vi "ABB change password.vi"() -> ()   [LabVIEW 2017]
uses:
  ABB global.vi
panel:
  out "Message":string
  in  "OK":bool
  in  "Cancel":bool
  in  "Confirm":string
  in  "New Password":string
  # "CHANGE PASSWORD"
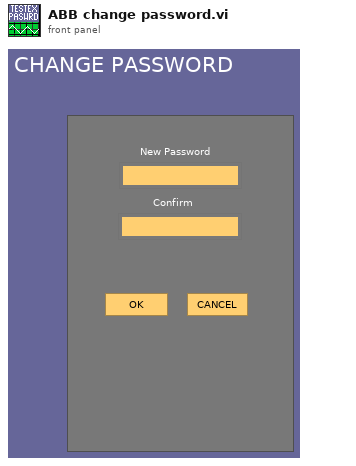
[diagram p1: front panel]
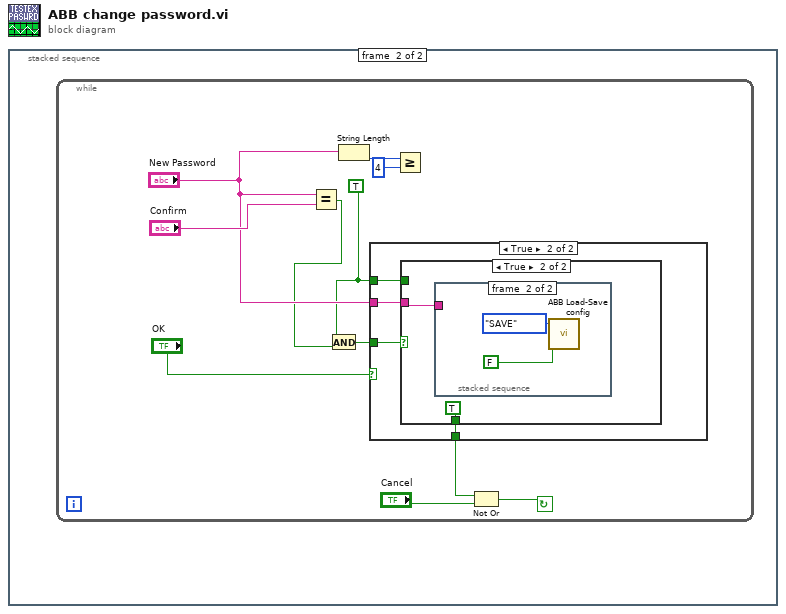
[diagram p0: block diagram]
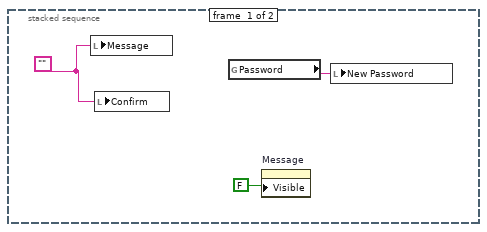
[diagram p2: hidden frame]
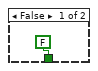
[diagram p3: hidden frame]
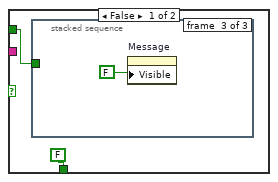
[diagram p4: hidden frame]
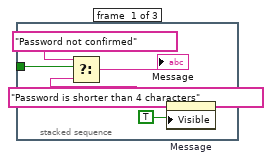
[diagram p5: hidden frame]
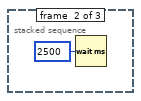
[diagram p6: hidden frame]
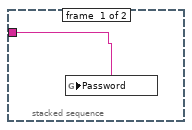
[diagram p7: hidden frame]
diagram:
  n1 = stacked-sequence {
    frame #0 {
      w2 = ""
      n2 = local write "Message"(w2) -> ()
      n3 = local write "Confirm"(w2) -> ()
      n4 = global read "ABB global.vi" "Password"() -> (w1:string)
      n5 = property on="Message" class="Str"("Visible"=FALSE ("Write Attribute")) -> ()  [unwired: 2 in, 2 out]
      n6 = local write "New Password"(w1) -> ()
    }
    frame #1 {
      n7 = while {
        stop <- w10 continue-if-true
        w4 = TRUE
        n8 = Equal?(x="New Password", y="Confirm") -> (x = y?=w7:bool)
        n9 = And(x=w4, y=w7) -> (x .and. y?=w6:bool)
        n10 = String Length(string="New Password") -> (length=w13:i32)
        n11 = case shown="True" "OK" {
          tunnel: "New Password" -> [_ w19]
          tunnel: w6 -> [_ w18]
          tunnel: [FALSE w17] -> w5
          tunnel: w4 -> [_ w16]
          frame False {
          }
          frame True {
            n12 = case shown="True" w18 {
              tunnel: w19 -> [_ w30]
              tunnel: [FALSE TRUE] -> w17
              tunnel: w16 -> [w20 _]
              frame False {
                n13 = stacked-sequence {
                  tunnel: w20 -> [w26 _ _]
                  frame #0 {
                    n14 = Select(t="Password not confirmed", s=w26, f="Password is shorter than 4 characters") -> (s? t:f=→"Message":string)
                    n15 = property on="Message" class="Str"("Visible"=TRUE ("Write Attribute")) -> ()  [unwired: 2 in, 2 out]
                  }
                  frame #1 {
                    n16 = Wait (ms)(milliseconds to wait=u32 2500) -> ()  [unwired: 1 out]
                  }
                  frame #2 {
                    n17 = property on="Message" class="Str"("Visible"=FALSE ("Write Attribute")) -> ()  [unwired: 2 in, 2 out]
                  }
                }
              }
              frame True {
                n18 = stacked-sequence {
                  tunnel: w30 -> [w31 _]
                  frame #0 {
                    n19 = global write "ABB global.vi" "Password"(w31) -> ()
                  }
                  frame #1 {
                    n20 = call "ABB Load-Save config.vi"("confirm save"=FALSE, "Mode"=enum16{"LOAD", "SAVE"}."SAVE") -> ()  [unwired: 10 in]
                  }
                }
              }
            }
          }
        }
        n21 = Greater Or Equal?(x=w13, y=4) -> ()  [unwired: 1 out]
        n22 = Not Or(1:"Cancel", 2:w5) -> (0:w10:bool)
      }
    }
  }
